vi "LabVIEW Datatype Prefix.vi"() -> (0 "datatype prefix":string="LVdatatype_")   [LabVIEW 2018]
panel:
  # "Prefix stored in this VI as default value."
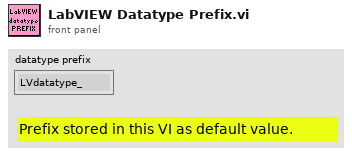
[diagram p1: front panel]
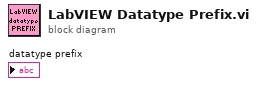
[diagram p0: block diagram]
diagram:
